vi "SetConfig.vi"(8 "error in (no error)":errorcluster, 10 "PARAM":string, 11 "Device in":refnum<class "Device.lvclass">) -> (0 "error out":errorcluster, 2 "RESP":string, 3 "Device out":refnum<class "Device.lvclass">)   [LabVIEW 2018, in "Device.lvclass"]
uses:
  Device.lvclass
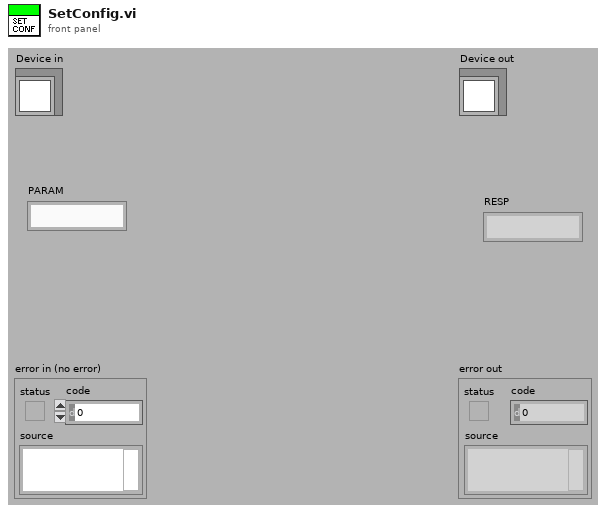
[diagram p1: front panel]
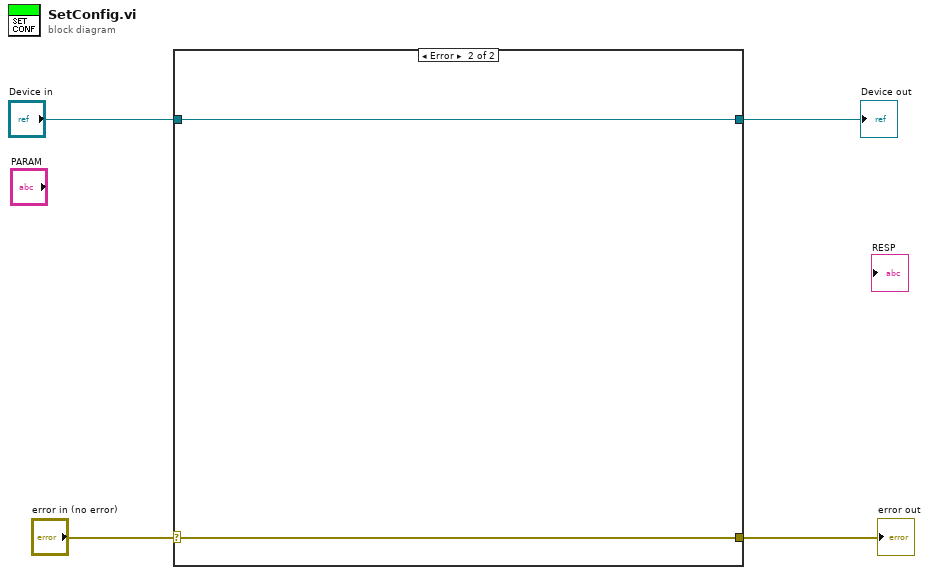
[diagram p0: block diagram]
diagram:
  n1 = case shown="Error" "error in (no error)" {
    selector: "error in (no error)" -> [w6 w8]
    tunnel: "Device in" -> [w5 w7]
    tunnel: [w6 w8] -> w2
    tunnel: [w5 w7] -> w1
    frame No Error {
    }
    frame Error {
    }
  }
  "error out" <- w2
  "Device out" <- w1
